vi "Project Login.vi"(0 "Enable":bool=TRUE caption="启用", 1 "厂区":u16(ring) items=["清溪", "松山湖"], 5 "error in (no error)":errorcluster caption="错误输入（无错误）") -> (12 "厂区":string, 16 "密码":string, 17 "用户名":string, 18 "登录":bool, 19 "error out":errorcluster caption="错误输出")   [LabVIEW 2011]
doc: "显示标准对话框，提示用户输入用户名、密码等信息。\n--------------------\n\n该Express VI配置如下:\n\n显示给用户的信息:VNA档案配置\n该输入为: \n文本输入框: 用户名\n文本输入框: 密码"
panel:
  in  "密码":string
  in  "用户名":string
  out "String":string="VNA档案配置" caption="字符串"
  in  "Cancel":bool caption="取消"
  in  "OK2":bool
  in  "OK1":bool
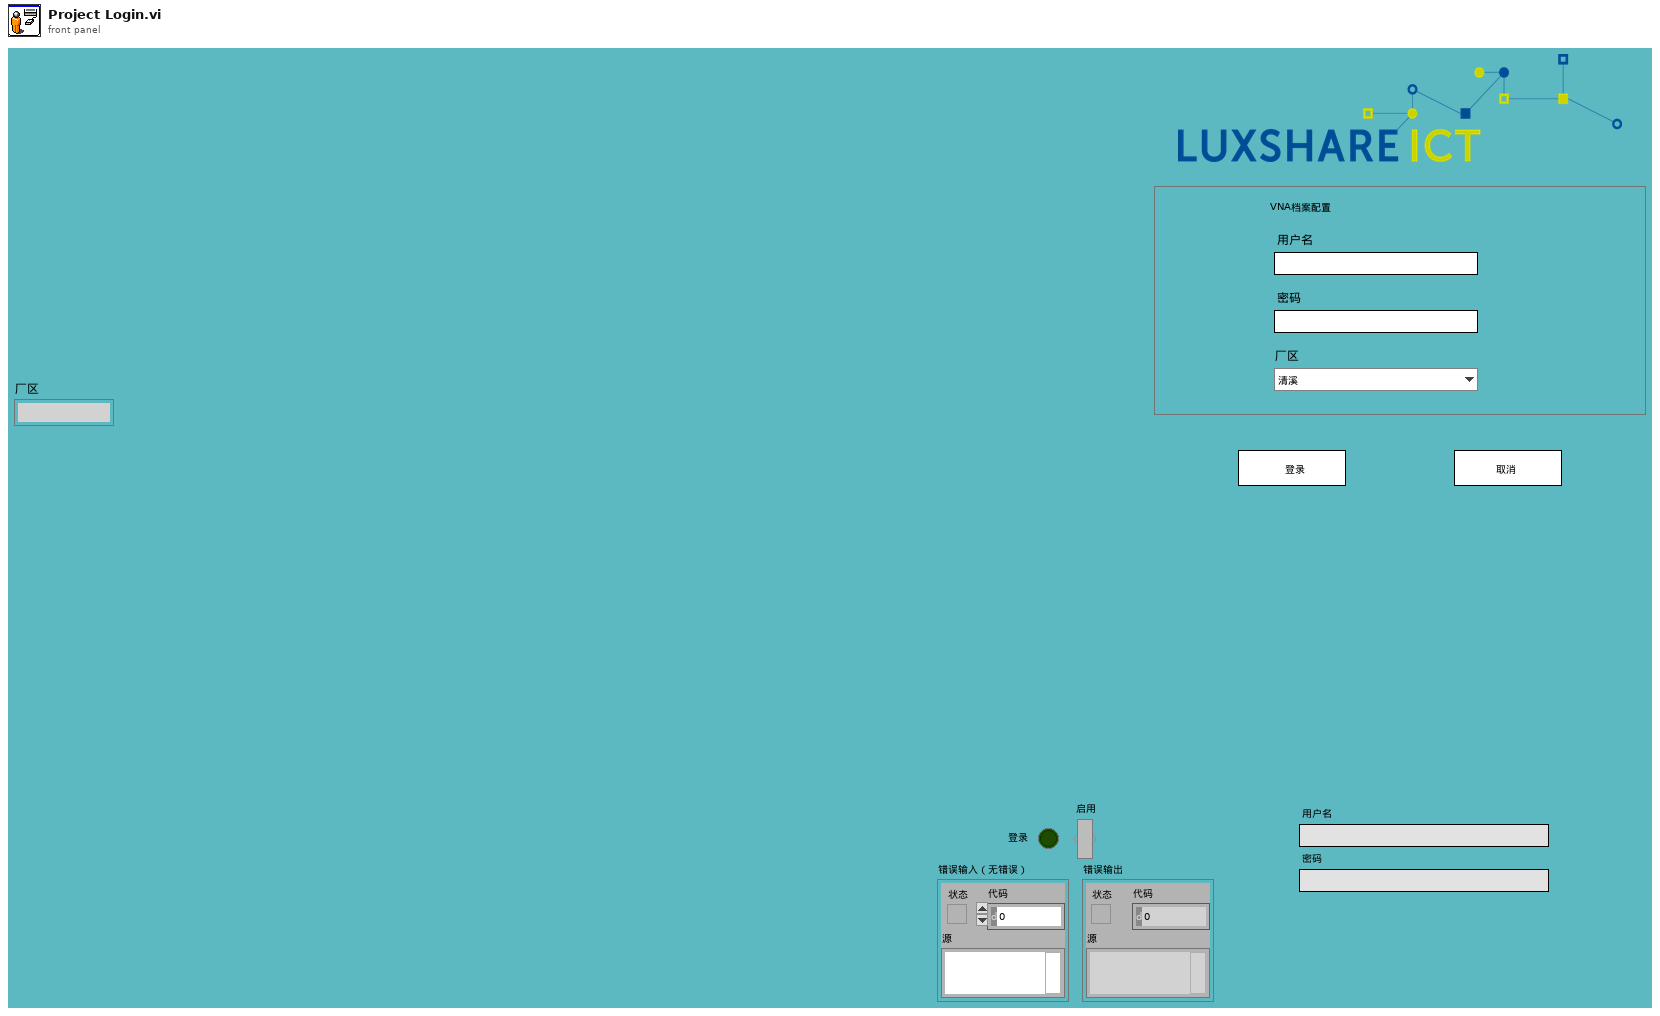
[diagram p1: front panel]
types:
  T1 = cluster{"Input Name":string, "Input Data Type":i32}[]
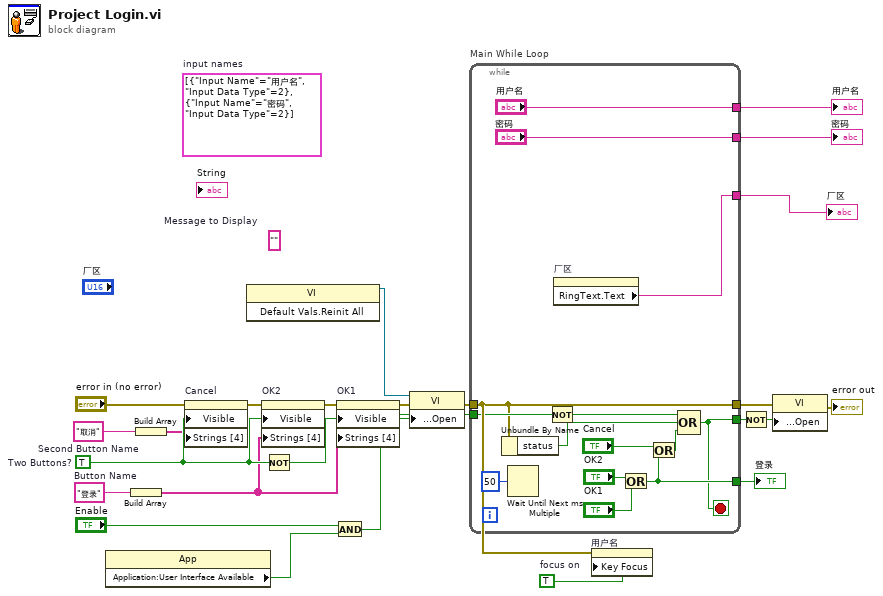
[diagram p0: block diagram]
diagram:
  w3 = TRUE  # focus on
  (unwired) T1 [{"Input Name"="用户名", "Input Data Type"=2}, {"Input Name"="密码", "Input Data Type"=2}]  # input names
  w16 = "取消"  # Second Button Name
  w14 = "登录"  # Button Name
  (unwired) ""  # Message to Display
  w24 = TRUE  # Two Buttons?
  n1 = property class="App"() -> ("Application:User Interface Available"=w6:bool)  [unwired: 2 in, 2 out]
  n2 = Build Array(w14) -> (w15:string[])
  n3 = Build Array(w16) -> (w17:string[])
  n4 = property on="Cancel" class="Bool"(error in="error in (no error)", "Visible"=w24, "Strings [4]"=w17) -> (error out=w21:errorcluster)  [unwired: 1 in, 1 out]
  n5 = invoke class="VI" method="Default Vals.Reinit All"() -> (reference out=w5:refnum<vi>)  [unwired: 3 in, 2 out]
  n6 = property on="OK2" class="Bool"(error in=w21, "Visible"=w24, "Strings [4]"=w15) -> (error out=w20:errorcluster)  [unwired: 1 in, 1 out]
  n7 = Not(x=w24) -> (.not. x?=w22:bool)
  n8 = And(x="Enable", y=w6) -> (x .and. y?=w7:bool)
  n9 = property on="OK1" class="Bool"(error in=w20, "Visible"=w22, "Strings [4]"=w15) -> (error out=w13:errorcluster)  [unwired: 1 in, 1 out]
  n10 = property class="VI"(reference=w5, error in=w13, "Front Panel Window:Open"=w7) -> (error out=w12:errorcluster)  [unwired: 1 out]
  n11 = while "Main While Loop" {
    tunnel: [w35] -> w23
    tunnel: w7 -> [w33]
    tunnel: [w31] -> w18
    tunnel: w12 -> [w30]
    tunnel: [w30] -> w10
    tunnel: ["用户名"] -> w4
    tunnel: ["密码"] -> w2
    tunnel: [w25] -> w1
    stop <- w31 stop-if-true
    n12 = Unbundle By Name(w30) -> ("status"=w28:bool)
    n13 = Wait Until Next ms Multiple(millisecond multiple=u32 50) -> ()  [unwired: 1 out]
    n14 = Not(x=w33) -> (.not. x?=w32:bool)
    n15 = property on="厂区" class="Ring (严格)"() -> ("RingText.Text"=w25:string)  [unwired: 2 in, 2 out]
    n16 = Or(x="OK2", y="OK1") -> (x .or. y?=w35:bool)
    n17 = Or(x="Cancel", y=w35) -> (x .or. y?=w29:bool)
    n18 = Compound Arithmetic op=OR(w32, w28, w29) -> (w31:bool)
  }
  "登录" <- w23
  "用户名" <- w4
  "密码" <- w2
  "厂区" <- w1
  n19 = property on="用户名" class="Str"(error in=w12, "Key Focus"=w3) -> ()  [unwired: 1 in, 2 out]
  n20 = Not(x=w18) -> (.not. x?=w19:bool)
  n21 = property class="VI"(error in=w10, "Front Panel Window:Open"=w19) -> (error out=→"error out":errorcluster)  [unwired: 1 in, 1 out]
